vi "Cancel Active Graphic On Click.vi"(8 "error in (no error)":errorcluster, 11 "Canvas in":refnum<class "Canvas.lvclass">) -> (0 "error out":errorcluster, 3 "Canvas out":refnum<class "Canvas.lvclass">)   [LabVIEW 2015, in "Canvas.lvclass"]
uses:
  Canvas.lvclass
  Graphic/Graphic.lvclass
  Canvas.lvclass/Canvas.ctl
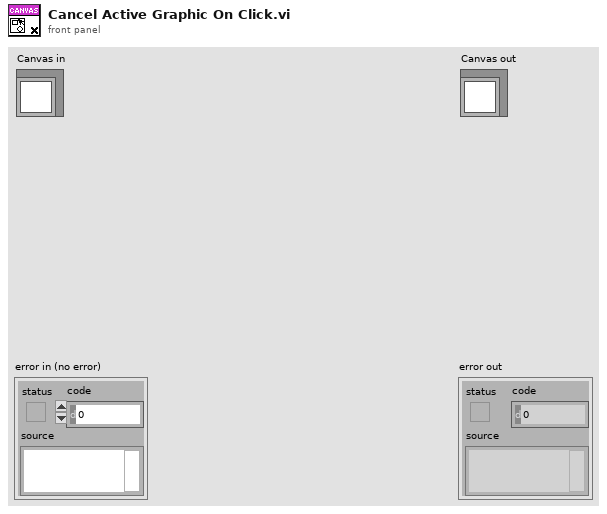
[diagram p1: front panel]
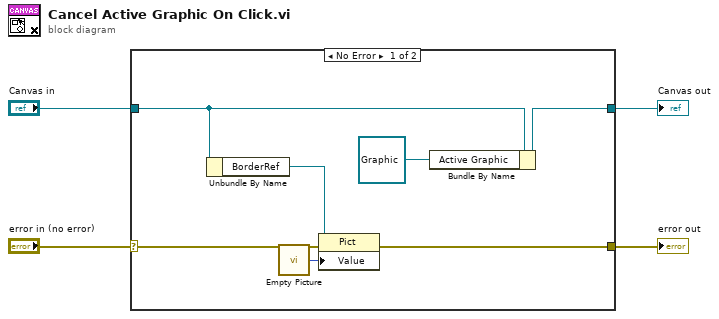
[diagram p0: block diagram]
diagram:
  n1 = case shown="No Error" "error in (no error)" {
    selector: "error in (no error)" -> [w10 w13]
    tunnel: [w7 w13] -> w3
    tunnel: [w6 w12] -> w1
    tunnel: "Canvas in" -> [w11 w12]
    frame No Error {
      n2 = Unbundle By Name(w11) -> ("BorderRef"=w9:refnum<vi>)
      n3 = call "Empty Picture"() -> ("empty picture"=w8:picture)
      n4 = property class="Pict"(reference=w9, error in=w10, "Value"=w8) -> (error out=w7:errorcluster)  [unwired: 1 out]
      n5 = Bundle By Name(cluster=w11, "Active Graphic"=refnum<class "Graphic.lvclass"> refnum ("Graphic.lvclass")) -> (w6:refnum<class "Canvas.lvclass">)
    }
    frame Error {
    }
  }
  "error out" <- w3
  "Canvas out" <- w1
